vi "CRYFlatten Serial No.vi"(11 "Serial#":T1) -> (3 "Serial# flattened":string)   [LabVIEW 2013]
uses:
  Typedef Control/CRYSerial No.ctl
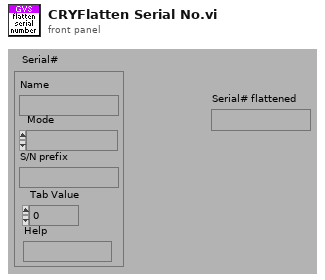
[diagram p1: front panel]
types:
  T1 = typedef "CRYSerial No.ctl" = cluster{"Name":string, "Mode":u16, "S/N prefix":string, "Tab Value":u16, "Help":string}
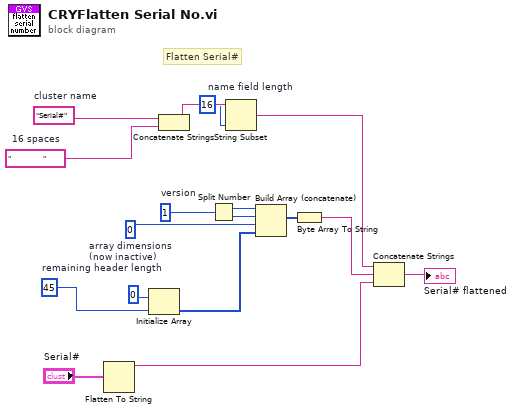
[diagram p0: block diagram]
diagram:
  w15 = u8 0  # array dimensions (now inactive)
  w12 = 16  # name field length
  w11 = "                "  # 16 spaces
  w10 = "Serial#"  # cluster name
  w5 = 45  # remaining header length
  w1 = u16 1  # version
  # "Flatten Serial#"
  n1 = Flatten To String(anything="Serial#") -> (data string=w17:string)  [unwired: 1 in, 4 out]
  n2 = Initialize Array(u8 0, w5) -> (w9:u8[])
  n3 = Concatenate Strings(w10, w11) -> (w13:string)
  n4 = Split Number(x=w1) -> (hi(x)=w2:u8, lo(x)=w3:u8)
  n5 = String Subset(string=w13, length (rest)=w12) -> (substring=w14:string)  [unwired: 1 out]
  n6 = Build Array (concatenate)(w2, w3, w15, w9) -> (w6:u8[])
  n7 = Byte Array To String(unsigned byte array=w6) -> (string=w8:string)
  n8 = Concatenate Strings(w14, w8, w17) -> (→"Serial# flattened":string)
